vi "Get all Alive GDs IDs.vi"(8 "error in (no error)":errorcluster, 11 "Guardian List in":refnum<class "Guardian List.lvclass">) -> (0 "error out":errorcluster, 2 "Alive GDs IDs":string[](array[string]), 3 "Guardian List out":refnum<class "Guardian List.lvclass">)   [LabVIEW 2026, in "TALOS.lvlib" / "Classes.lvlib" / "Guardian List.lvclass"]
uses:
  Guardian List.lvclass
  Guardian List.lvclass/Guardian List.ctl
  71aebf99-3c91-4249-bd95-3adf7cf6b129.vi
  <vilib>/Comparison/Less/Less Functor/Less Functor.lvclass
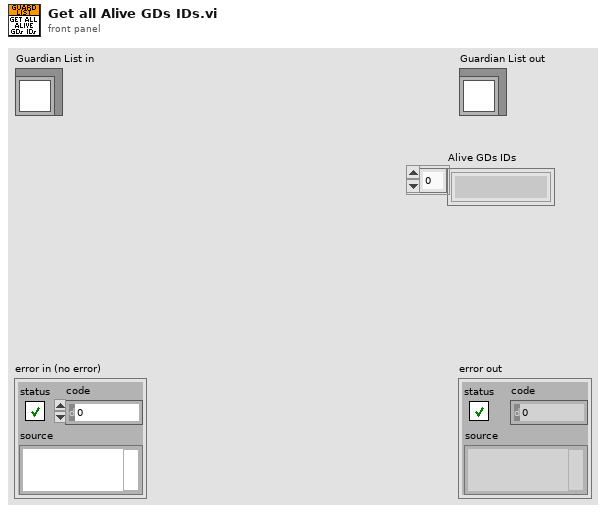
[diagram p1: front panel]
types:
  T1 = typedef "TALOS.lvlib/Classes.lvlib/Guardian List.lvclass/Guardian Properties.ctl" = cluster{"Alive":bool, "Last Seen":timestamp, "IP":string, "TCP Writer associated ID":string, "uS List received":bool, "Abort":bool, "Bearer":bool, "TCP Listener associated ID":string}
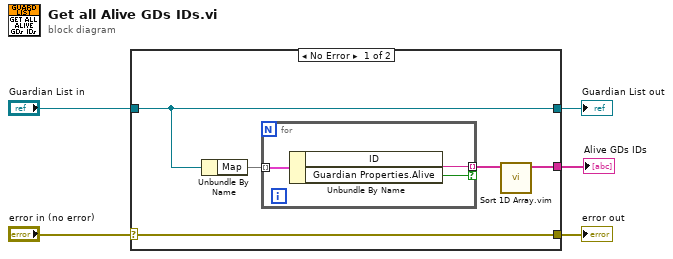
[diagram p0: block diagram]
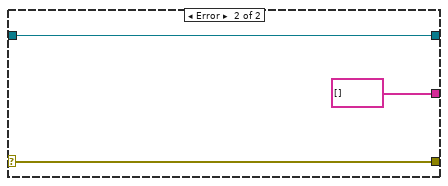
[diagram p2: hidden frame]
diagram:
  n1 = case shown="No Error" "error in (no error)" {
    selector: "error in (no error)" -> [w10 w16]
    tunnel: [w10 w16] -> w4
    tunnel: [w9 w15] -> w2
    tunnel: "Guardian List in" -> [w9 w15]
    tunnel: [w6 string[] []] -> w1
    frame No Error {
      n2 = Unbundle By Name(w9) -> ("Map"=w8:map{string, T1})
      n3 = for {
        tunnel: w8 -> [w13] mode=indexing
        tunnel: [w12] -> w7 mode=indexing if=w11
        n4 = Unbundle By Name(w13) -> ("ID"=w12:string, "Guardian Properties.Alive"=w11:bool)
      }
      n5 = call "Sort 1D Array.vim"("unsorted array"=w7) -> ("sorted array"=w6:string[])  [unwired: 10 in]
    }
    frame Error {
    }
  }
  "error out" <- w4
  "Guardian List out" <- w2
  "Alive GDs IDs" <- w1
